vi "LoadMenu.vi"(8 "error in (no error)":errorcluster, 11 "Game in":refnum<class "Game.lvclass">) -> (0 "error out":errorcluster, 3 "Game out":refnum<class "Game.lvclass">)   [LabVIEW 2019, in "RT_Game.lvlib" / "Game.lvclass"]
uses:
  Game.lvclass
  Menu/Menu.lvclass
  Game.lvclass/Game.ctl
  Write SwitchGame.vi
  Write FlattenedNextClass.vi
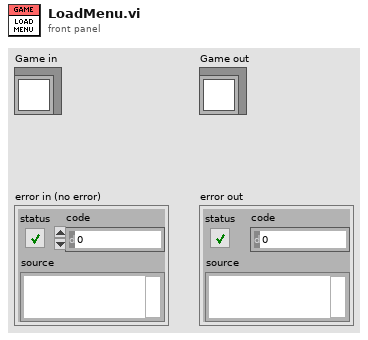
[diagram p1: front panel]
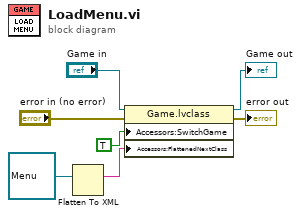
[diagram p0: block diagram]
diagram:
  n1 = Flatten To XML(anything=refnum<class "Menu.lvclass"> refnum ("RT_Game.lvlib:Menu.lvclass")) -> (xml string=w5:string)
  n2 = property class="Game.lvclass"(reference="Game in", error in="error in (no error)", "Accessors:SwitchGame"=TRUE ("SwitchGame_"), "Accessors:FlattenedNextClass"=w5) -> (reference out=→"Game out":refnum<class "Game.lvclass">, error out=→"error out":errorcluster)
